vi "FGV Stoerungen aufnehmen.vi"(6 "FGV Störung aufnehmen Aktion":T1, 10 "Störung ein":bool, 11 "Meldungs-Nummer":i32) -> (0 "quittieren?":bool, 1 "abschalten":bool, 2 "warnen":bool, 3 "aktive Störungen":bool[](array[boolean]))   [LabVIEW 2020, in "Stoerungen.lvlib"]
uses:
  Stoerungen.lvlib
  FGV Stoerung aufnehmen Aktion.ctl
  FGV Stoerungsdatei Aktionen.ctl
  FGV Stoermeldungen Aktion.ctl
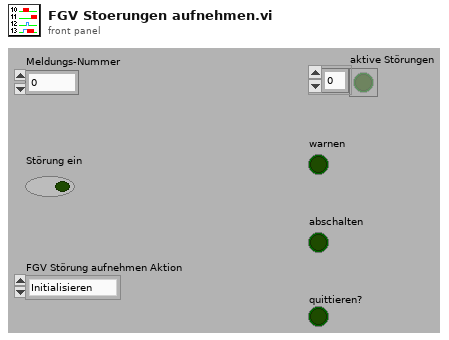
[diagram p1: front panel]
types:
  T1 = typedef "Stoerungen.lvlib/FGV Stoerung aufnehmen Aktion.ctl" = enum16{"Initialisieren", "Schreiben", "Lesen", "Quittieren", "quit. löschen"}
  T2 = typedef "Stoerungen.lvlib/FGV Stoerungsdatei Aktionen.ctl" = enum16{"lesen", "laden", "Neue Werte"}
  T3 = typedef "Stoerungen.lvlib/FGV Stoermeldungen Aktion.ctl" = enum16{"Initialisieren", "kommend", "gehend", "lesen", "Queue leeren", "Queue freigeben", "in Datei loggen", "Änderung zurücksetzen"}
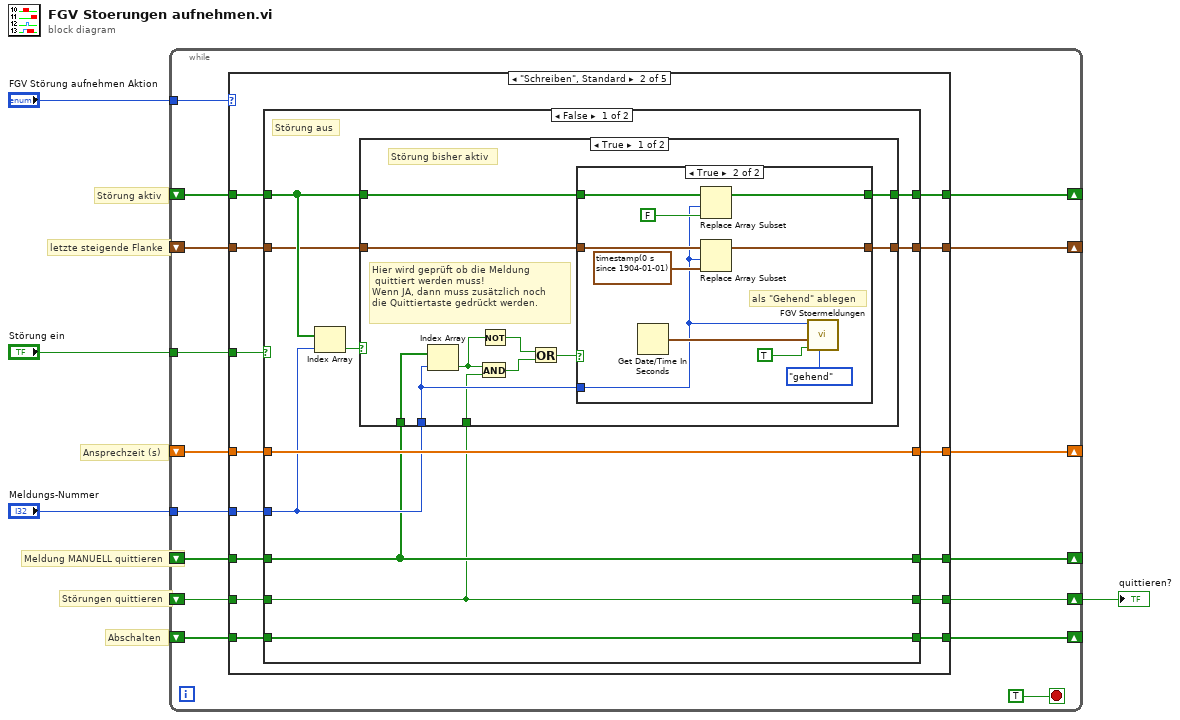
[diagram p0: block diagram]
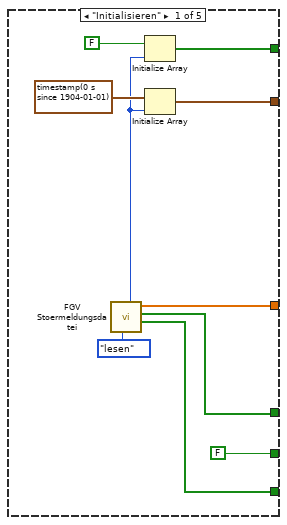
[diagram p2: hidden frame]
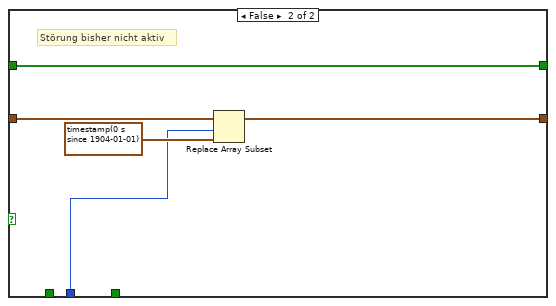
[diagram p4: hidden frame]
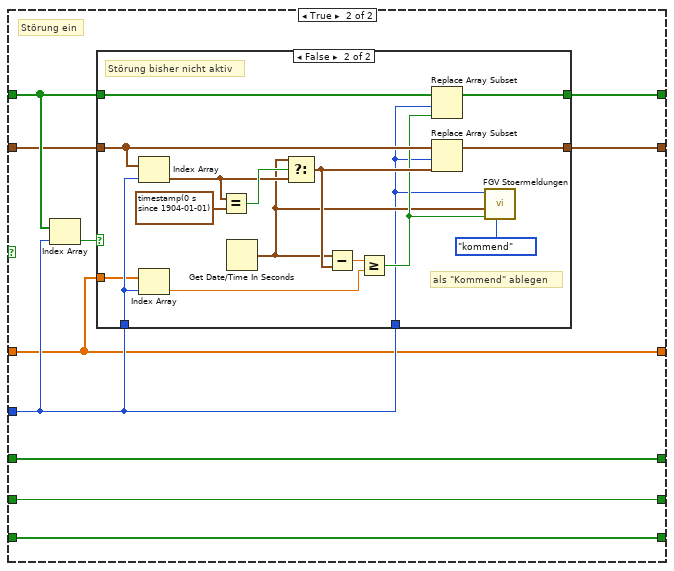
[diagram p5: hidden frame]
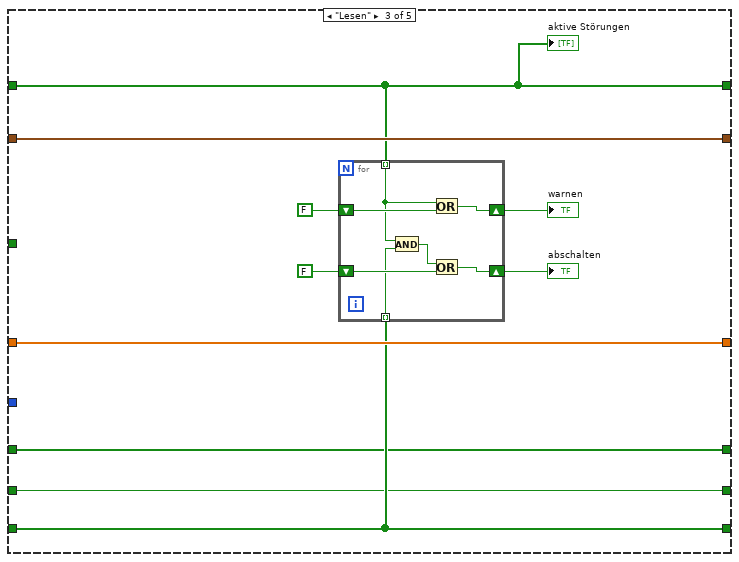
[diagram p7: hidden frame]
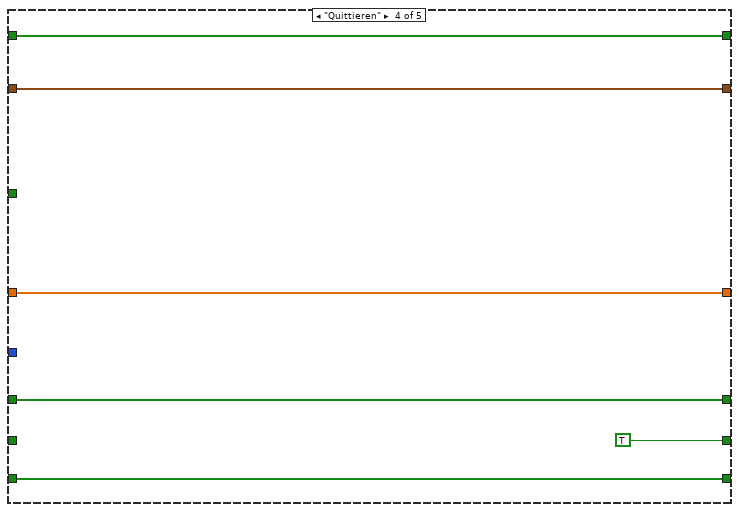
[diagram p8: hidden frame]
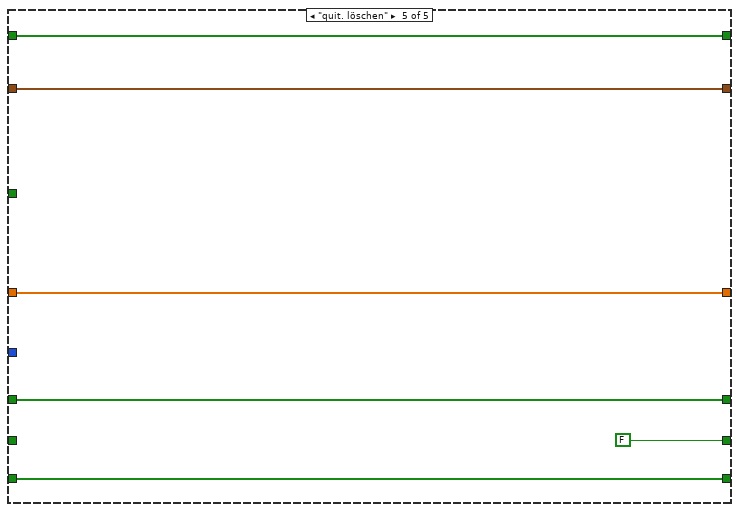
[diagram p9: hidden frame]
diagram:
  # "Meldung MANUELL quittieren"
  # "Störungen quittieren"
  # "Störung aktiv"
  # "letzte steigende Flanke"
  # "Ansprechzeit (s)"
  # "Abschalten"
  n1 = while {
    shift-right: [w19] -> _
    shift-left: _ -> [w16]
    tunnel: "FGV Störung aufnehmen Aktion" -> [w20]
    shift-right: [w18] -> _
    shift-left: _ -> [w15]
    shift-right: [w17] -> _
    shift-left: _ -> [w14]
    shift-right: [w12] -> _
    shift-left: _ -> [w11]
    tunnel: "Störung ein" -> [w10]
    tunnel: "Meldungs-Nummer" -> [w9]
    shift-right: [w5] -> w1
    shift-left: _ -> [w6]
    shift-right: [w8] -> _
    shift-left: _ -> [w7]
    stop <- TRUE stop-if-true
    n2 = case shown="\"Schreiben\", Standard" w20 {
      tunnel: [w29 w36 w116 w133 w139] -> w19
      tunnel: [w28 w37 w120 w132 w138] -> w18
      tunnel: [w24 w40 w119 w131 w137] -> w17
      tunnel: w16 -> [_ w43 w116 w133 w139]
      tunnel: w15 -> [_ w42 w120 w132 w138]
      tunnel: w14 -> [_ w41 w119 w131 w137]
      tunnel: [w25 w38 w115 w130 w136] -> w12
      tunnel: w11 -> [_ w39 w115 w130 w136]
      tunnel: w10 -> [_ w44 _ _ _]
      tunnel: w9 -> [_ w35 _ _ _]
      tunnel: [FALSE w34 w112 TRUE FALSE] -> w5
      tunnel: w6 -> [_ w31 w112 _ _]
      tunnel: [w22 w32 w111 w128 w134] -> w8
      tunnel: w7 -> [_ w33 w111 w128 w134]
      frame "Initialisieren" {
        n3 = call "FGV Stoermeldungsdatei.vi"("Aktionen"=FGV_Stoerungsdatei_Aktionen."lesen") -> ("abschaltend"=w25:bool[], "quittieren?"=w22:bool[], "Ansprechverzögerung"=w24:dbl[], "max Nummer"=w26:i32)  [unwired: 2 in, 5 out]
        n4 = Initialize Array(FALSE, w26) -> (w29:bool[])
        n5 = Initialize Array(timestamp(0 s since 1904-01-01), w26) -> (w28:timestamp[])
      }
      frame "Schreiben", Default {
        n6 = case shown="False" w44 {
          tunnel: w43 -> [w51 w90]
          tunnel: w42 -> [w48 w87]
          tunnel: w41 -> [w53 w85]
          tunnel: [w53 w85] -> w40
          tunnel: w39 -> [w54 w92]
          tunnel: [w54 w92] -> w38
          tunnel: [w50 w89] -> w37
          tunnel: [w49 w88] -> w36
          tunnel: w35 -> [w47 w86]
          tunnel: w31 -> [w45 w84]
          tunnel: [w45 w84] -> w34
          tunnel: w33 -> [w46 w83]
          tunnel: [w46 w83] -> w32
          frame False {
            # "Störung aus"
            n7 = Index Array(array=w51, index=w47) -> (element=w52:bool)
            n8 = case shown="True" w52 {
              tunnel: w51 -> [w62 w79]
              tunnel: [w65 w82] -> w50
              tunnel: [w64 w79] -> w49
              tunnel: w48 -> [w63 w81]
              tunnel: w47 -> [w60 w78]
              tunnel: w46 -> [w61 _]
              tunnel: w45 -> [w59 _]
              frame True {
                # "Hier wird geprüft ob die Meldung\n quittiert werden muss!\nWenn JA, dann muss zusätzlich noch \ndie Quittiertaste gedrückt werden."
                # "Störung bisher aktiv"
                n9 = Index Array(array=w61, index=w60) -> (element=w55:bool)
                n10 = And(x=w55, y=w59) -> (x .and. y?=w57:bool)
                n11 = Not(x=w55) -> (.not. x?=w56:bool)
                n12 = Or(x=w56, y=w57) -> (x .or. y?=w58:bool)
                n13 = case shown="True" w58 {
                  tunnel: [w66 w77] -> w65
                  tunnel: [w67 w76] -> w64
                  tunnel: w63 -> [w66 w75]
                  tunnel: w62 -> [w67 w74]
                  tunnel: w60 -> [_ w68]
                  frame False {
                  }
                  frame True {
                    # "als \"Gehend\" ablegen"
                    n14 = Get Date/Time In Seconds() -> (seconds since 1Jan1904=w70:timestamp)
                    n15 = Replace Array Subset(array=w74, new element=FALSE, index=w68) -> (w76:bool[])
                    n16 = Replace Array Subset(array=w75, new element=timestamp(0 s since 1904-01-01), index=w68) -> (w77:timestamp[])
                    n17 = call "FGV Stoermeldungen.vi"("Aktion"=FGV_Stoermeldungen_Aktion."gehend", "eintragen"=TRUE, "Zeitstempel"=w70, "Meldungs-Nummer"=w68) -> ()  [unwired: 1 in, 7 out]
                  }
                }
              }
              frame False {
                # "Störung bisher nicht aktiv"
                n18 = Replace Array Subset(array=w81, new element=timestamp(0 s since 1904-01-01), index=w78) -> (w82:timestamp[])
              }
            }
          }
          frame True {
            # "Störung ein"
            n19 = Index Array(array=w90, index=w86) -> (element=w91:bool)
            n20 = case shown="False" w91 {
              tunnel: w90 -> [w93 w100]
              tunnel: [w94 w110] -> w89
              tunnel: [w93 w99] -> w88
              tunnel: w87 -> [w94 w109]
              tunnel: w86 -> [_ w95]
              tunnel: w86 -> [_ w103]
              tunnel: w85 -> [_ w102]
              frame True {
                # "Störung bisher aktiv"
              }
              frame False {
                # "als \"Kommend\" ablegen"
                # "Störung bisher nicht aktiv"
                n21 = Index Array(array=w109, index=w103) -> (element=w106:timestamp)
                n22 = Index Array(array=w102, index=w103) -> (element=w101:dbl)
                n23 = Equal?(x=w106, y=timestamp(0 s since 1904-01-01)) -> (x = y?=w107:bool)
                n24 = Get Date/Time In Seconds() -> (seconds since 1Jan1904=w96:timestamp)
                n25 = Select(t=w96, s=w107, f=w106) -> (s? t:f=w105:timestamp)
                n26 = Subtract(x=w96, y=w105) -> (x-y=w104:dbl)
                n27 = Greater Or Equal?(x=w104, y=w101) -> (x >= y?=w97:bool)
                n28 = Replace Array Subset(array=w100, new element=w97, index=w95) -> (w99:bool[])
                n29 = Replace Array Subset(array=w109, new element=w105, index=w95) -> (w110:timestamp[])
                n30 = call "FGV Stoermeldungen.vi"("Aktion"=FGV_Stoermeldungen_Aktion."kommend", "eintragen"=w97, "Zeitstempel"=w96, "Meldungs-Nummer"=w95) -> ()  [unwired: 1 in, 7 out]
              }
            }
          }
        }
      }
      frame "Lesen" {
        n31 = for {
          shift-right: [w126] -> w114
          shift-left: FALSE -> [w127]
          shift-right: [w121] -> w113
          shift-left: FALSE -> [w125]
          tunnel: w116 -> [w123] mode=indexing
          tunnel: w115 -> [w122] mode=indexing
          n32 = And(x=w123, y=w122) -> (x .and. y?=w124:bool)
          n33 = Or(x=w123, y=w127) -> (x .or. y?=w126:bool)
          n34 = Or(x=w124, y=w125) -> (x .or. y?=w121:bool)
        }
        "warnen" <- w114
        "abschalten" <- w113
        "aktive Störungen" <- w116
      }
      frame "Quittieren" {
      }
      frame "quit. löschen" {
      }
    }
  }
  "quittieren?" <- w1
